vi "save ITC log.vi"(6 "action":enum16{"init", "check"}(ring)=enum."check", 7 "file path":path=path "E:/Data/spagetti/18_to20K_feb13", 8 "temperature boxes":T1={"LTC21 Address"="GPIB0::15::INSTR", "ITC503 Address"="GPIB0::24::INSTR", "ITC temperature"=74.95, "ITC set temperature"=72.62, "LTC temperature"=87.267, "heater"=0.1, "gas flow"=12.2, "P"=21.91, "D"=0.1, "I"=1.2, "ITC state"="X0A1C2S01H1L0\r", "nonzero temperature"=87.267, "Magn Field (T)"=0.0, "LakeShore340"="GPIB0::16::INSTR", "LS340 Adress"=16, "Sample Temperature Source"=enum."read T <- LakeShore 340", "Neocera sensor"=1}, 9 "seconds":dbl=8971.4, 11 "save log":T3={"file path"=path "E:/Data/spagetti/18_to20K_feb13", "Save log?"=TRUE, "every # of sec"=30}) -> (1 "saving log to":string, 3 "save log out":T3={"file path"=path "E:/Data/spagetti/18_to20K_feb13", "Save log?"=TRUE, "every # of sec"=30})   [LabVIEW 2015]
uses:
  save log.ctl
  state.ctl
  Sample_Temperature_Source_Control.ctl
  ctl -- name dispatcher -- action.ctl
  Q -- check range -- i -- real.vi
  Q - not nan and gtr than zero - Real.vi
  file -- 9w path.vi
  Q - not nan -- real.vi
  <vilib>/Utility/libraryn.llb/Check if File or Folder Exists.vi
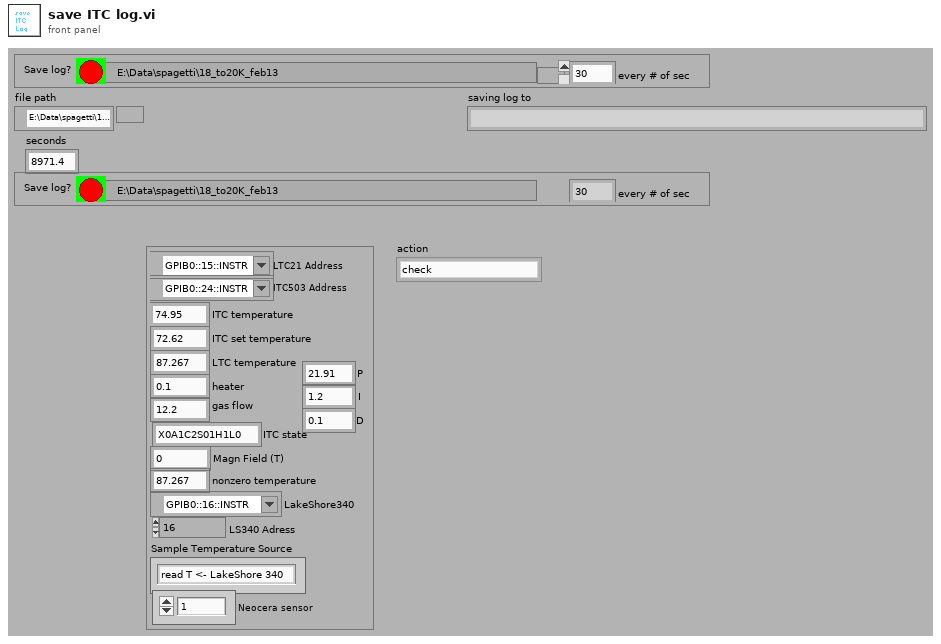
[diagram p1: front panel]
types:
  T1 = typedef "state.ctl" = cluster{"LTC21 Address":refnum<visa-resource-name>, "ITC503 Address":refnum<visa-resource-name>, "ITC temperature":dbl, "ITC set temperature":dbl, "LTC temperature":dbl, "heater":dbl, "gas flow":dbl, "P":dbl, "D":dbl, "I":dbl, "ITC state":string, "nonzero temperature":dbl, "Magn Field (T)":dbl, "LakeShore340":refnum<visa-resource-name>, "LS340 Adress":i16, "Sample Temperature Source":T2, "Neocera sensor":i32}
  T2 = typedef "Sample_Temperature_Source_Control.ctl" = enum16{"read T <- LakeShore 340", "read T <- Neocera"}
  T3 = typedef "save log.ctl" = cluster{"file path":path, "Save log?":bool, "every # of sec":i32}
  T4 = typedef "ctl -- name dispatcher -- action.ctl" = enum16{"peak frequency", "peak frequency DUMP", "peak gamma DUMP", "peak gamma", "peak frequency TEST", "peak gamma TEST", "ultrasonic power", "time in gamma", "set temperature ", "set temperature timer", "peak default gamma", "last scan file", "peak freq gamma TEST", "peak NAMES", "errors", "P_I_D", "P", "I", "D", "power vs time", "power vs time TIMER", "void", "power log", "set temperature - SINE", "itc ltc log", "peak - time in gamma"}
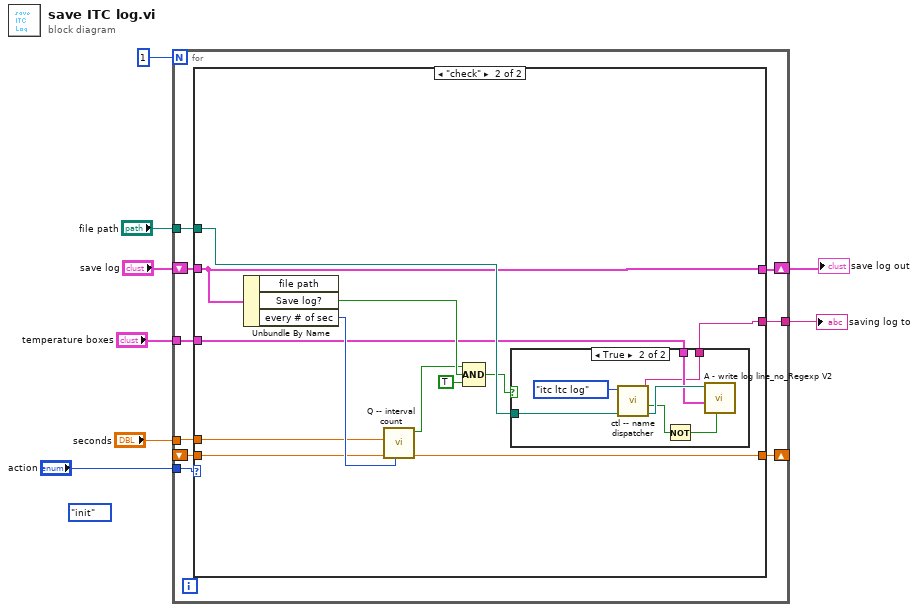
[diagram p0: block diagram]
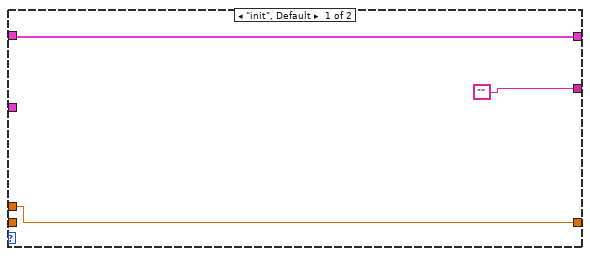
[diagram p2: hidden frame]
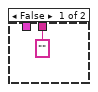
[diagram p3: hidden frame]
diagram:
  (unwired) enum16{"init", "check"}."init" ("disable interaction with itc")
  n1 = for {
    N: 1 -> [_]
    tunnel: "seconds" -> [w9]
    tunnel: "file path" -> [w16]
    tunnel: "temperature boxes" -> [w15]
    shift-right: [w14] -> w2
    shift-left: "save log" -> [w17]
    tunnel: [w13] -> w3
    shift-right: [w12] -> _
    shift-left: _ -> [w10]
    tunnel: "action" -> [w11]
    n2 = case shown="\"check\"" w11 {
      tunnel: w17 -> [w19 w23]
      tunnel: w16 -> [_ w26]
      tunnel: w15 -> [_ w25]
      tunnel: [w19 w23] -> w14
      tunnel: ["" w21] -> w13
      tunnel: [w18 w29] -> w12
      tunnel: w10 -> [_ w28]
      tunnel: w9 -> [w18 w27]
      frame "init", Default {
      }
      frame "check" {
        n3 = Unbundle By Name(w23) -> ("Save log?"=w32:bool, "every # of sec"=w30:i32)  [unwired: 1 out]
        n4 = call "Q -- interval count.vi"("interval (sec)"=w30, "last time (sec)"=w28, "current time (sec)"=w27) -> ("last time out (sec)"=w29:dbl, "tic"=w31:bool)  [unwired: 5 in, 2 out]
        n5 = Compound Arithmetic op=AND(w31, w32, TRUE ("value")) -> (w22:bool)
        n6 = case shown="True" w22 {
          tunnel: w26 -> [_ w40]
          tunnel: w25 -> [_ w37]
          tunnel: ["" ("ctl file name") w34] -> w21
          frame False {
          }
          frame True {
            n7 = call "ctl -- name dispatcher.vi"("sweep folder path"=w40, "ctl name dispatch"=ctl_--_name_dispatcher_--_action."itc ltc log") -> ("file path"=w38:path, "file or folder exists?"=w36:bool, "ctl file name"=w34:string)  [unwired: 7 in]
            n8 = Not(x=w36) -> (.not. x?=w35:bool)
            n9 = call "A - write log line_no_Regexp V2.vi"("file is new?"=w35, "temperature boxes"=w37, "file Path"=w38) -> ()  [unwired: 9 in]
          }
        }
      }
    }
  }
  "save log out" <- w2
  "saving log to" <- w3
